vi "Keithley 6485.vi"(0 "VISA resource name":refnum<visa-resource-name>="COM1", 1 "Baud Rate":u32=9600, 4 "Data Bits":u16=8 min=5 max=8 step=1, 5 "Parity":u16(ring) items=["None", "Odd", "Even", "Mark", "Space"], 7 "Stop Bits":u16(ring)=10 items=["1.0"=10, "1.5"=15, "2.0"=20], 9 "XON Character":u8=17 format="%.0x", 14 "XOFF Character":u8=19 format="%.0x", 15 "Timeout (ms)":u32=10000, 21 "End read on termination character?":bool=TRUE, 24 "Termination Char\n(0xA = '\\n' = LF)":u8=10 format="%.0x") -> ()   [LabVIEW 2010]
doc: "The Advanced Serial Read and Write example performs a Serial Port Read, a Serial Port Write, or a combination of these actions while setting some advanced serial features like buffer size, termination characters, and XON/XOFF flow control. The user selects the actions (read or write) on the front panel. If both are selected, the VI will write the data first, read the data and then close the VISA session that is opened to the port. \n\nThe parameters set for the serial port must match the parameters of the connected instrument or device. In this example, the bytes to read parameter specifies the number of bytes that the serial port reads. If there were more bytes at the port than the number specified in bytes to read, those bytes would not be read. Also, if you specify to read more bytes than the number of bytes actually read, you might receive a timeout error message.\n\nINSTRUCTIONS:\n1) Select the serial resource and configuration parameters (baud rate, data bits, parity, stop bits, flow control).\n2) Termination character can be enabled and set. Also, set the required input buffer size prior to running the example.\n3) Select the operations to be performed. \n4) Connect the serial port to your device. If no device is available, perform a loopback test by doing one of the following. Short pins 2 and 3 on a RS-232 cable or short pin 4 to pin 8 and pin 5 to pin 9 on a RS-485/422 cable. \n5) Run the VI to see the data read. (The \"read string\" will match the \"string to write\" if a loopback test was performed.)\n\nThis example exposes several advanced features that you may need for your application. Not all applications need all the features shown in this example. The input buffer size is likely an important setting that you want to control in your application. This example expands upon the flow control option for XON and XOFF, allowing the user to choose those control characters. The timeout parameter has been brought to the front panel so a user can specify the time period the VISA Read will wait for the number of bytes to read before timing out. Also, the user has several controls for the termination character, which is discussed later.\n\nNote that you can press the write and read buttons and change the bytes to read parameters on the fly, while the example is running. However, you must stop the example to change the other configuration parameters after the example has started running, and then run again.\n\nSet the I/O buffer size slightly higher the amount of data you expect to receive. This is very important for applications that don't use flow control, as you may lose characters if the receive buffer overflows.\n\nSetting the timeout period ensures that the operation returns with a timeout error if the operation cannot be performed in the specified time period. \n\nSome devices require a termination character in order to identify the end of command strings. Some devices send a termination character to signify the end of data to be read. \n\nThis example shows how you can end the Read operation once a termination character is detected in the buffer and/or append a termination character at the end of the Write data. To enable the Read to end on a termination character, use the VISA Configure Serial Port or use the VISA Properties Serial End Mode for Reads, Termination Character Enable, and Termination Character. To end the Write with a termination character, use the VISA Properties Serial End Mode for Writes, the Send End Enable, and Termination Character. In this example, the same termination character is used for both the Read and the Write. You can specify two different characters for your application, if desired.\n\nYour application may require specific characters for the XON/XOFF Flow Control. You can specify these characters with the VISA Properties Flow Control XOFF Character and Flow Control XON Character. Note that if the standard XON and XOFF characters are used, then decimal 17 and 19 are unavailable for data values. Remember that using flow control and setting an adequate buffer size allow you to prevent buffer overflows."
uses:
  <vilib>/Instr/_visa.llb/VISA Configure Serial Port (Instr).vi
  <vilib>/Analysis/NI_AALBase.lvlib
panel:
  out "read buffer":string
  in  "Tab Control":T1(tab)
  out "Error Has Occurred":bool
  out "Active":bool
  in  "Enable":bool
  out "Faraday Cup (A)":dbl
  in  "Error In":bool=TRUE
  in  "Flow Control":u16(ring) items=["None"=0, "XON/XOFF"=1, "RTS/CTS"=2, "DTR/DSR"=4]
  in  "Bytes to Read":i32
  in  "Error Procedure":string="SYST:ZCH OFF"
  in  "Initial Configuration":string="*RST"
  in  "Range Limits":string="SYST:ZCH OFF"
  in  "Enable Range Limits":bool
  in  "Samples":u32 min=1 max=2500
  out "Code":i32
  out "Source":string
  out "Message":string
  out "Error":string
  # "The first 9 commands are executed, in order, before any measurements are taken.\n\nNote that using all caps and short-form commands run faster.  See manual for more details."
  # "To begin taking measurements, flip the switch up.  Manual control of the picoammeter is disabled while measurements are being taken.  Flip the switch back down to stop measuring.  Maunal control is resumed when the 'Config/Local' button is pressed on the picoammeter."
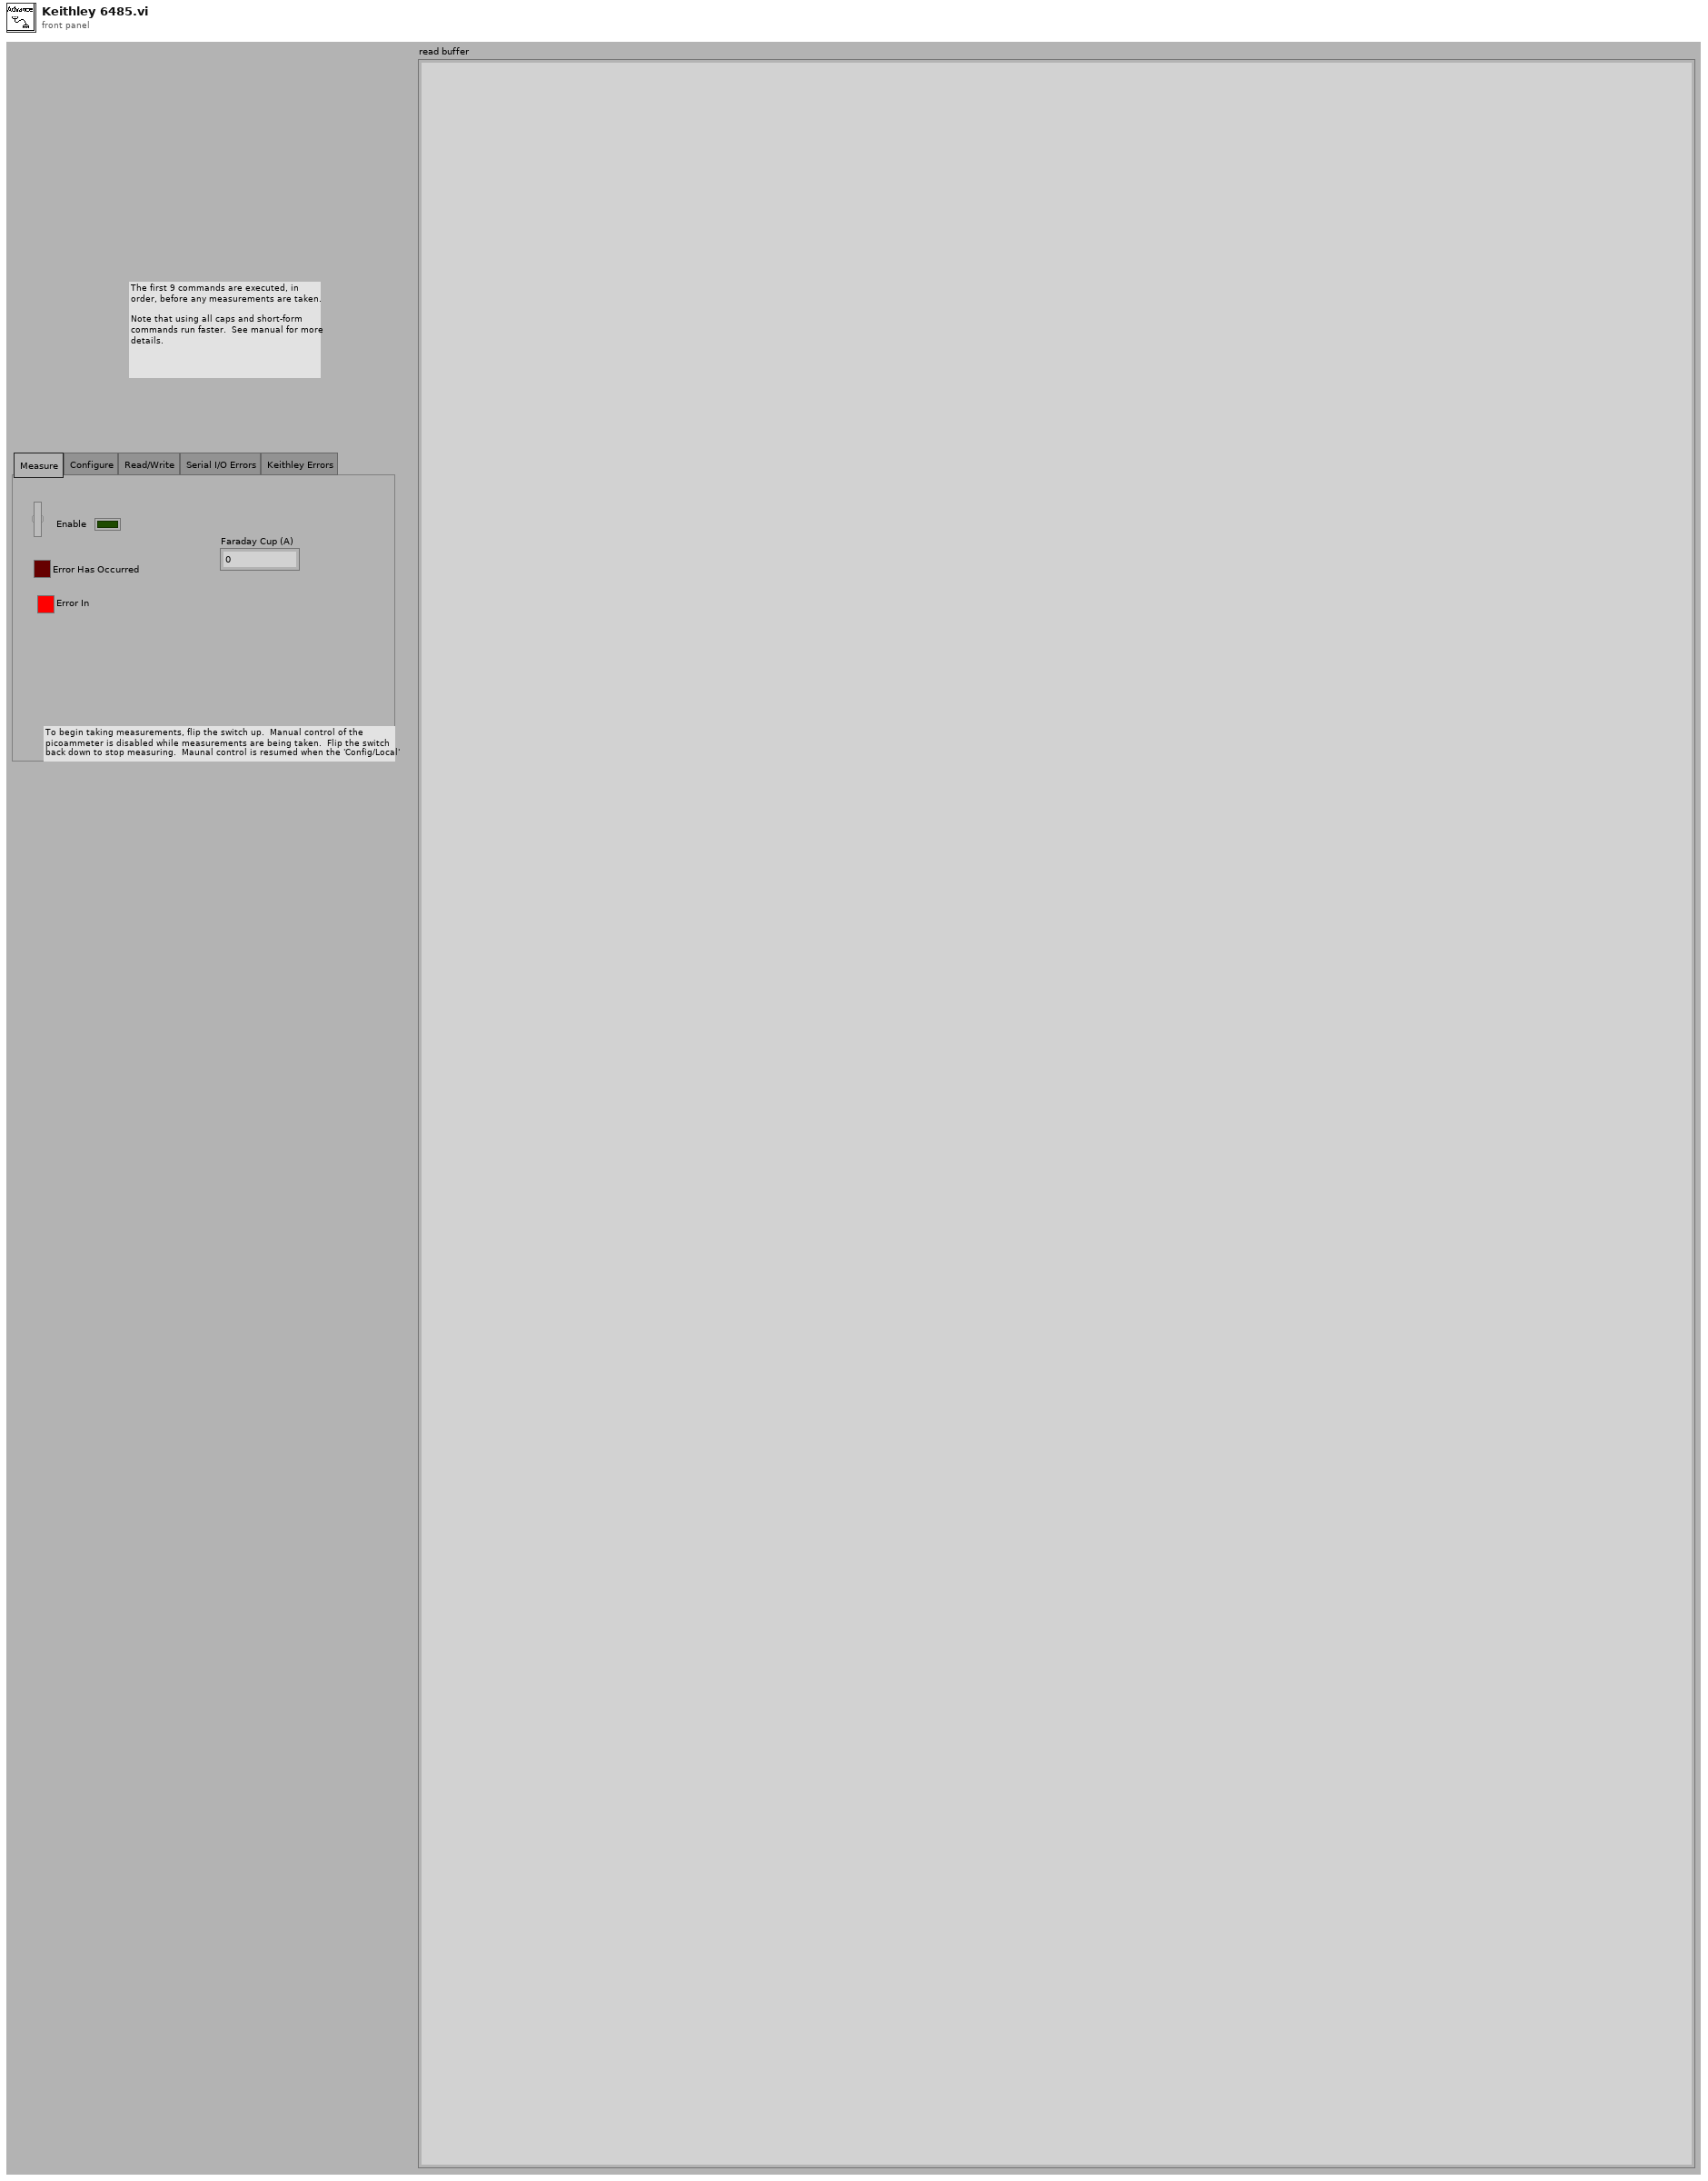
[diagram p1: front panel]
types:
  T1 = enum32{"Measure", "Configure", "Read/Write", "Serial I/O Errors", "Keithley Errors"}
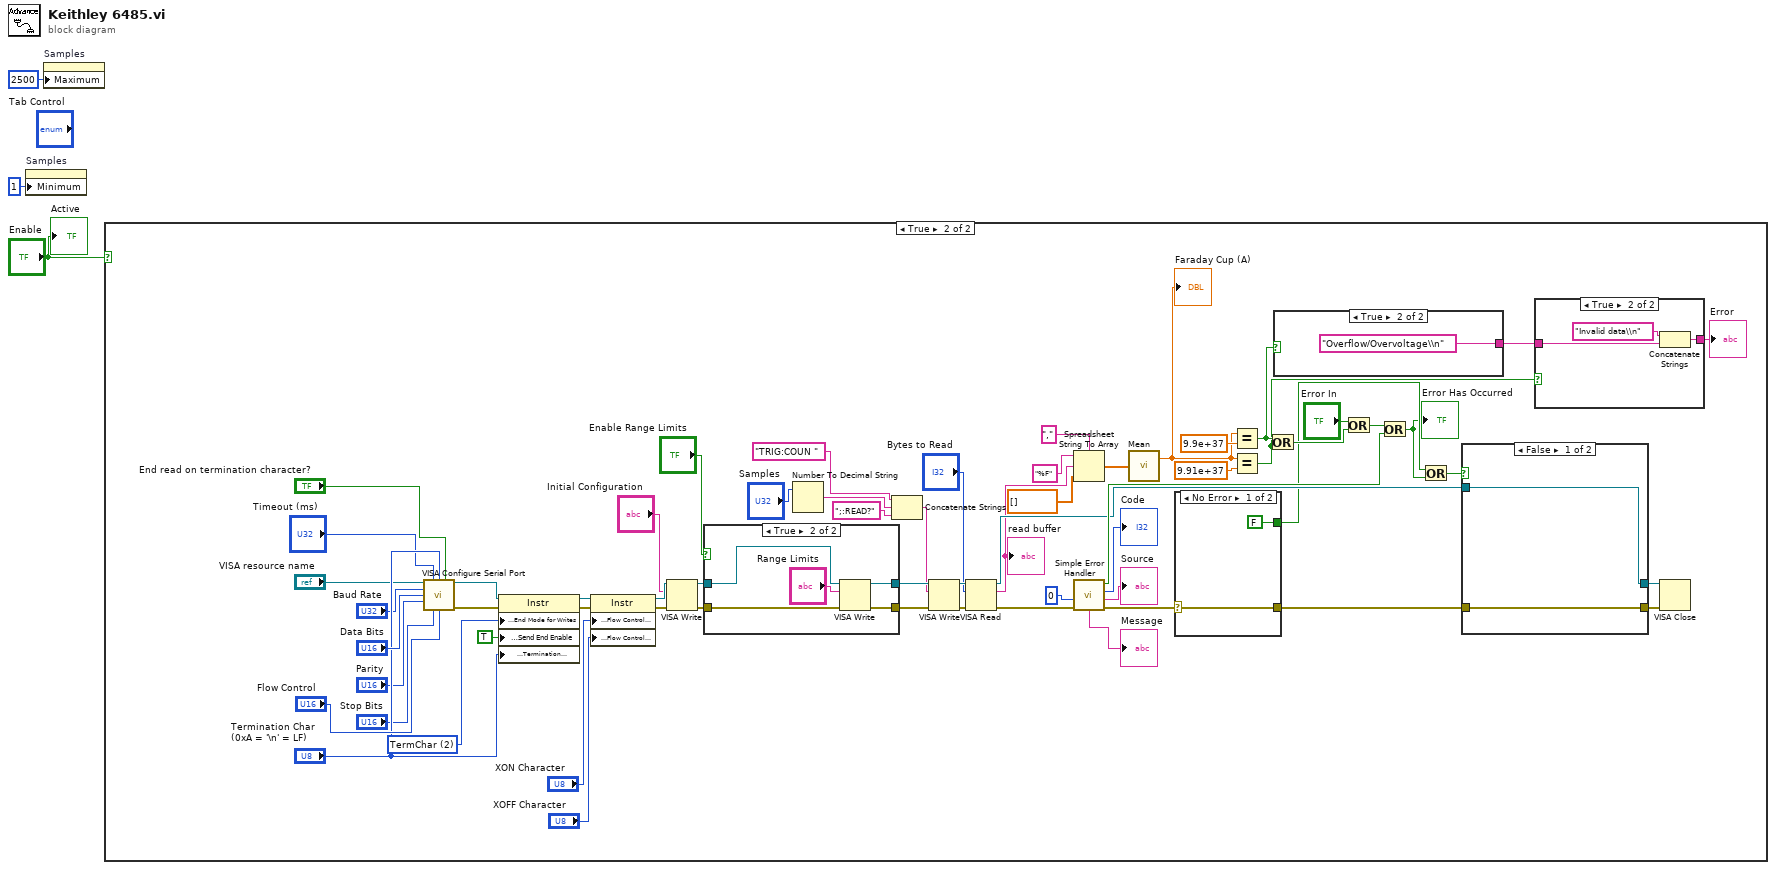
[diagram p0: block diagram]
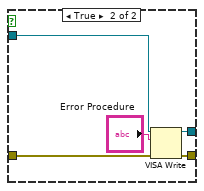
[diagram p3: hidden frame]
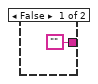
[diagram p5: hidden frame]
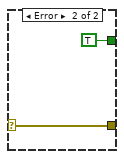
[diagram p7: hidden frame]
diagram:
  n1 = property on="Samples" class="DigNum (strict)"("Minimum"=1) -> ()  [unwired: 2 in, 2 out]
  n2 = property on="Samples" class="DigNum (strict)"("Maximum"=2500) -> ()  [unwired: 2 in, 2 out]
  n3 = case shown="True" "Enable" {
    frame False {
    }
    frame True {
      w62 = u16 2 items=["None", "LastBit", "TermChar", "Break"] ("Serial Settings:Serial End Mode for Writes")
      n4 = call-poly "VISA Configure Serial Port"("VISA resource name"="VISA resource name", "timeout (10sec)"="Timeout (ms)", "termination char\n(0xA = '\\n' = LF)"="Termination Char\n(0xA = '\\n' = LF)", "Enable Termination\nChar (T)"="End read on termination character?", "baud rate (9600)"="Baud Rate", "data bits (8)"="Data Bits", "parity (0:none)"="Parity", "stop bits (10: 1 bit)"="Stop Bits", "flow control (0:none)"="Flow Control") -> ("VISA resource name out"=w61:refnum<visa-resource-name>, "error out"=w60:errorcluster)  [unwired: 1 in, 4 out]
      n5 = property on="Property Node" class="Instr"(reference=w61, error in=w60, "Serial Settings:End Mode for Writes"=w62, "Message Based Settings:Send End Enable"=TRUE, "Message Based Settings:Termination Character"="Termination Char\n(0xA = '\\n' = LF)") -> (reference out=w64:refnum<visa-resource-name>, error out=w65:errorcluster)
      n6 = property class="Instr"(reference=w64, error in=w65, "Serial Settings:Flow Control XON Character"="XON Character", "Serial Settings:Flow Control XOFF Character"="XOFF Character") -> (reference out=w50:refnum<visa-resource-name>, error out=w49:errorcluster)
      n7 = VISA Write(VISA resource name=w50, write buffer="Initial Configuration", error in (no error)=w49) -> (VISA resource name out=w47:refnum<visa-resource-name>, error out=w46:errorcluster)  [unwired: 1 out]
      n8 = case shown="True" "Enable Range Limits" {
        tunnel: w47 -> [w80 w85]
        tunnel: w46 -> [w79 w84]
        tunnel: [w80 w83] -> w30
        tunnel: [w79 w82] -> w31
        frame False {
        }
        frame True {
          n9 = VISA Write(VISA resource name=w85, write buffer="Range Limits", error in (no error)=w84) -> (VISA resource name out=w83:refnum<visa-resource-name>, error out=w82:errorcluster)  [unwired: 1 out]
        }
      }
      n10 = Number To Decimal String(number="Samples") -> (decimal integer string=w14:string)  [unwired: 1 in]
      n11 = Concatenate Strings("TRIG:COUN ", w14, ";:READ?") -> (w13:string)
      n12 = VISA Write(VISA resource name=w30, write buffer=w13, error in (no error)=w31) -> (VISA resource name out=w28:refnum<visa-resource-name>, error out=w29:errorcluster)  [unwired: 1 out]
      n13 = VISA Read(VISA resource name=w28, byte count="Bytes to Read", error in (no error)=w29) -> (VISA resource name out=w25:refnum<visa-resource-name>, read buffer=w8:string, error out=w40:errorcluster)  [unwired: 1 out]
      "read buffer" <- w8
      n14 = Spreadsheet String To Array(delimiter (Tab)=",", format string="%F", spreadsheet string=w8, array type (2D Dbl)=dbl[] [] ("Array")) -> (array=w5:dbl[])
      n15 = call <vilib>:"Simple Error Handler.vi"("type of dialog (OK msg:1)"=0, "error in (no error)"=w40) -> ("error?"=w39:bool, "code out"=→"Code":i32, "source out"=→"Source":string, "error out"=w26:errorcluster, "message"=→"Message":string)  [unwired: 3 in]
      n16 = call <vilib>:"Mean.vi"("X"=w5) -> ("mean"=w4:dbl)  [unwired: 1 out]
      "Faraday Cup (A)" <- w4
      n17 = case shown="No Error" w26 {
        selector: w26 -> [w87 w89]
        tunnel: [w87 w89] -> w24
        tunnel: [FALSE TRUE] -> w21
        frame No Error {
        }
        frame Error {
        }
      }
      n18 = Equal?(x=w4, y=9.9e+37) -> (x = y?=w38:bool)
      n19 = Equal?(x=w4, y=9.91e+37) -> (x = y?=w37:bool)
      n20 = Or(x=w38, y=w37) -> (x .or. y?=w34:bool)
      n21 = case shown="True" w38 {
        tunnel: ["" "Overflow/Overvoltage\\n"] -> w36
        frame False {
        }
        frame True {
        }
      }
      n22 = Or(x="Error In", y=w34) -> (x .or. y?=w32:bool)
      n23 = Or(x=w32, y=w39) -> (x .or. y?=w20:bool)
      "Error Has Occurred" <- w20
      n24 = Or(x=w21, y=w20) -> (x .or. y?=w19:bool)
      n25 = case shown="False" w19 {
        tunnel: w25 -> [w67 w71]
        tunnel: w24 -> [w66 w70]
        tunnel: [w67 w69] -> w23
        tunnel: [w66 w68] -> w22
        frame False {
        }
        frame True {
          n26 = VISA Write(VISA resource name=w71, write buffer="Error Procedure", error in (no error)=w70) -> (VISA resource name out=w69:refnum<visa-resource-name>, error out=w68:errorcluster)  [unwired: 1 out]
        }
      }
      n27 = case shown="True" w37 {
        tunnel: w36 -> [w73 w76]
        tunnel: [w73 w74] -> w35
        frame False {
        }
        frame True {
          n28 = Concatenate Strings("Invalid data\\n", w76) -> (w74:string)
        }
      }
      "Error" <- w35
      n29 = VISA Close(VISA resource name=w23, error in (no error)=w22) -> ()  [unwired: 1 out]
    }
  }
  "Active" <- "Enable"
